vi "jog stop.vi"(8 "error in (no error)":errorcluster, 11 "Stepper in":refnum<class "Stepper.lvclass">) -> (0 "error out":errorcluster, 3 "Stepper out":refnum<class "Stepper.lvclass">)   [LabVIEW 2025, in "Stepper.lvclass"]
uses:
  Stepper.lvclass
  Stepper.lvclass/Stepper.ctl
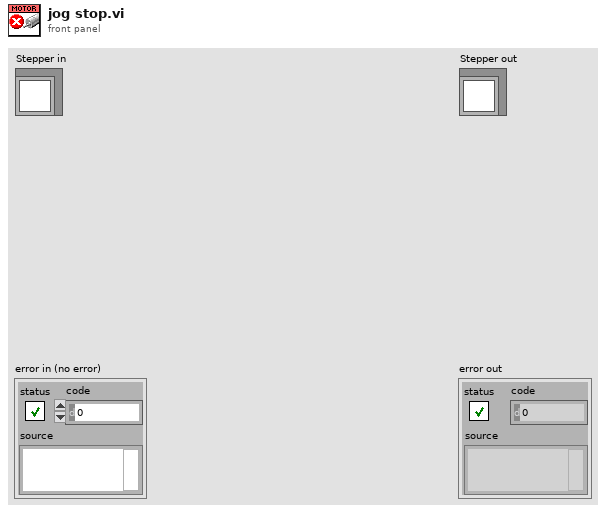
[diagram p1: front panel]
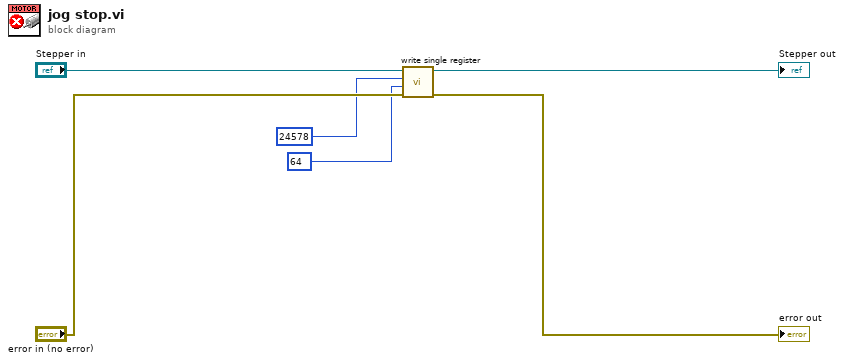
[diagram p0: block diagram]
diagram:
  n1 = call-dynamic "write single register.vi"("error in (no error)"="error in (no error)", "register to write"=u16 64 ("address"), "address"=u16 24578, "Stepper in"="Stepper in") -> ("error out"=→"error out":errorcluster, "Stepper out"=→"Stepper out":refnum<class "Stepper.lvclass">)  [unwired: 6 in]
